vi "Timer.vi"() -> (1 "time":bool, 2 "Wait Time out":u32)   [LabVIEW 2015]
uses:
  Control PB/timer.ctl
  Control Button/Exit.ctl
panel:
  in  "Exit":T1
  in  "Wait Time":u32=100 caption="Timer(ms)" max=600000 step=1
  in  "Timer":T2
  # "Delay (ms)"
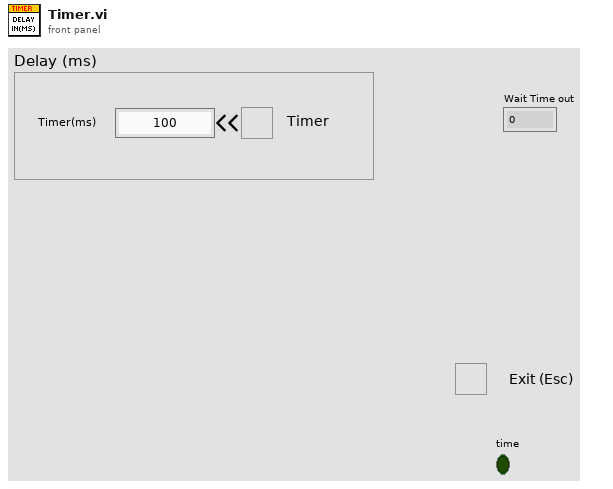
[diagram p1: front panel]
types:
  T1 = typedef "Exit.ctl" = bool
  T2 = typedef "timer.ctl" = bool
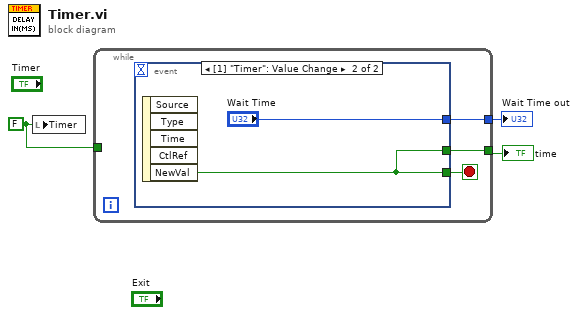
[diagram p0: block diagram]
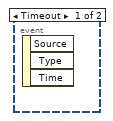
[diagram p2: hidden frame]
diagram:
  w2 = T2 FALSE ("Timer")
  n1 = local write "Timer"(w2) -> ()
  n2 = while {
    tunnel: [w5] -> w3
    tunnel: w2 -> [_]
    tunnel: [w4] -> w1
    stop <- w6 stop-if-true
    n3 = event shown="[1] \"Timer\": Value Change" {
      selector: _ -> [_ _]
      dyn-events: _ -> [_ _]
      timeout: _ -> [_ _]
      tunnel: [_ w7] -> w6
      tunnel: [_ "Wait Time"] -> w5
      tunnel: [_ w7] -> w4
      event Timeout {
        n4 = event-data() -> ()  [unwired: 1 in, 3 out]
      }
      event Value Change {
        n5 = event-data() -> ("NewVal"=w7:T2)  [unwired: 1 in, 4 out]
      }
    }
  }
  "Wait Time out" <- w3
  "time" <- w1
